vi "Set Domain.vi"(8 "error in (no error)":errorcluster, 10 "domain":variant, 11 "Domain_Evolut_2D_Rect in":refnum<class "NI_Domain_Evolut_2D_Rect.lvclass">) -> (0 "error out":errorcluster, 3 "Domain_Evolut_2D_Rect out":refnum<class "NI_Domain_Evolut_2D_Rect.lvclass">)   [LabVIEW 2017, in "NI_PDE.lvlib" / "NI_Domain_Evolut_2D_Rect.lvclass"]
uses:
  <vilib>/gmath/pde.llb/DomainClass/Domain_Evolut_2D_Rect/NI_Domain_Evolut_2D_Rect.lvclass
  <vilib>/gmath/pde.llb/DomainClass/Domain_Evolut_2D_Rect/Domain Data.ctl
  <vilib>/gmath/pde.llb/DomainClass/Domain_Evolut_2D_Rect/NI_Domain_Evolut_2D_Rect.lvclass/NI_Domain_Evolut_2D_Rect.ctl
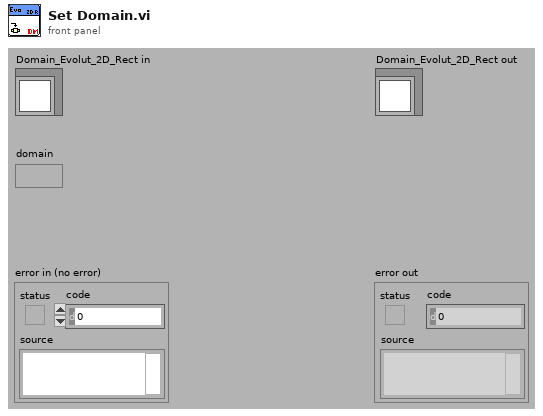
[diagram p1: front panel]
types:
  T1 = typedef "NI_PDE.lvlib/NI_Domain_Evolut_2D_Rect.lvclass/Domain Data.ctl" = cluster{"T":cluster{"initial t":dbl, "final t":dbl, "# of t-points":i32}, "X":cluster{"start x":dbl, "end x":dbl, "# of x-points":i32}, "Y":cluster{"start y":dbl, "end y":dbl, "# of y-points":i32}}
  T2 = cluster{"start x":dbl, "end x":dbl, "# of x-points":i32}
  T3 = cluster{"start y":dbl, "end y":dbl, "# of y-points":i32}
  T4 = cluster{"initial t":dbl, "final t":dbl, "# of t-points":i32}
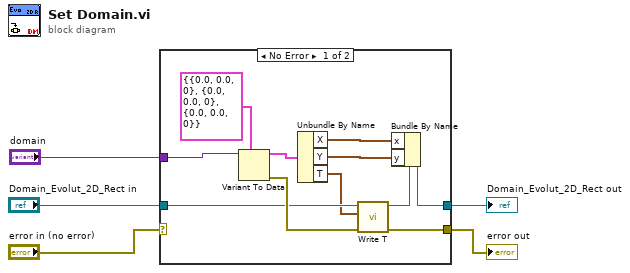
[diagram p0: block diagram]
diagram:
  n1 = case shown="No Error" "error in (no error)" {
    selector: "error in (no error)" -> [_ w18]
    tunnel: "Domain_Evolut_2D_Rect in" -> [w11 w17]
    tunnel: [w6 w17] -> w5
    tunnel: [w14 w18] -> w4
    tunnel: "domain" -> [w16 _]
    frame No Error {
      n2 = Variant To Data(type=T1 {"T"={"initial t"=0.0, "final t"=0.0, "# of t-points"=0}, "X"={"start x"=0.0, "end x"=0.0, "# of x-points"=0}, "Y"={"start y"=0.0, "end y"=0.0, "# of y-points"=0}} ("domain data"), Variant=w16) -> (data=w13:T1, error out=w15:errorcluster)  [unwired: 1 in]
      n3 = Unbundle By Name(w13) -> ("X"=w10:T2, "Y"=w9:T3, "T"=w8:T4)
      n4 = call-dynamic "Write T.vi"("error in (no error)"=w15, "t"=w8, "Domain_Evolut.lvclass in"=w11) -> ("error out"=w14:errorcluster, "Domain_Evolut.lvclass out"=w7:refnum<class "NI_Domain_Evolut_2D_Rect.lvclass">)  [unwired: 7 out]
      n5 = Bundle By Name(cluster=w7, "x"=w10, "y"=w9) -> (w6:refnum<class "NI_Domain_Evolut_2D_Rect.lvclass">)
    }
    frame Error {
    }
  }
  "Domain_Evolut_2D_Rect out" <- w5
  "error out" <- w4
